vi "Create a simple numeric vi.vi"   [LabVIEW 2012]
uses:
  <vilib>/Utility/miscctls.llb/LVPointTypeDef.ctl
  <vilib>/Utility/miscctls.llb/LVBoundsTypeDef.ctl
  Scripting Tools.lvlib
types:
  T1 = typedef "LVPointTypeDef.ctl" = cluster{"Horizontal":i16, "Vertical":i16}
  T2 = typedef "LVBoundsTypeDef.ctl" = cluster{"Width":u32, "Height":u32}
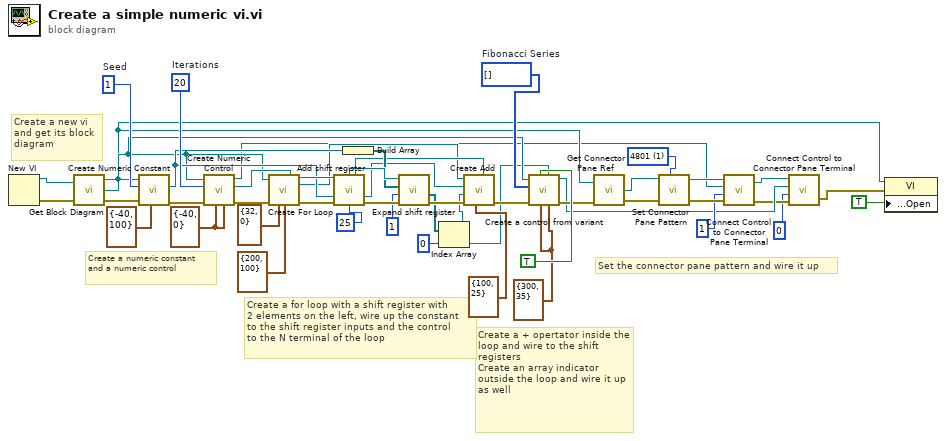
[diagram p0: block diagram]
diagram:
  w10 = u16 1 items=["4800", "4801", "4802", "4803", "4804", "4805", "4806", "4807", "4808", "4809", "4810", "4811", "4812", "4813", "4814", "4815", "4816", "4817", "4818", "4819", "4820", "4821", "4822", "4823", "4824", "4825", "4826", "4827", "4828", "4829", "4830", "4831", "4832", "4833", "4834", "4835"] ("Pattern")
  w19 = i32[] []  # Fibonacci Series
  w15 = T1 {"Horizontal"=300, "Vertical"=35} ("relative position/next to refnum")
  w16 = T1 {"Horizontal"=-40, "Vertical"=0} ("relative position/next to refnum")
  w46 = 20  # Iterations
  w43 = 1  # Seed
  # "Set the connector pane pattern and wire it up"
  # "Create a + opertator inside the loop and wire to the shift registers\nCreate an array indicator outside the loop and wire it up as well"
  # "Create a for loop with a shift register with\n2 elements on the left, wire up the constant\nto the shift register inputs and the control\nto the N terminal of the loop"
  # "Create a numeric constant\nand a numeric control"
  # "Create a new vi\nand get its block\ndiagram"
  n1 = New VI() -> (0:w47:errorcluster, 3:w48:refnum<vi>)  [unwired: 1 in, 6 out]
  n2 = call "Get Block Diagram.vi"("vi refnum in"=w48, "error in (no error)"=w47) -> ("Diagram"=w18:refnum<vi>, "vi refnum out"=w13:refnum<vi>, "error out"=w45:errorcluster)
  n3 = call "Create Numeric Constant.vi"("relative position/next to refnum"=T1 {"Horizontal"=-40, "Vertical"=100}, "error in (no error)"=w45, "Value"=w43, "Diagram"=w18) -> ("error out"=w44:errorcluster, "Output Terminal"=w32:refnum<vi>)  [unwired: 1 in, 5 out]
  n4 = call "Create Numeric Control.vi"("Terminal Position"=w16, "FP Position"=w16, "error in (no error)"=w44, "Value"=w46, "Diagram"=w18) -> ("error out"=w41:errorcluster, "Output Terminal"=w20:refnum<vi>, "Control Ref"=w7:refnum<vi>)  [unwired: 2 in, 2 out]
  n5 = call "Create For Loop.vi"("Diagram In"=w18, "Loop Count Source"=w20, "error in (no error)"=w41, "relative position/next to refnum"=T1 {"Horizontal"=32, "Vertical"=0}, "Frame Size"=T2 {"Width"=200, "Height"=100}) -> ("For Loop ref"=w37:refnum<vi>, "Diagram"=w24:refnum<vi>, "error out"=w38:errorcluster)  [unwired: 3 in, 5 out]
  n6 = call "Add shift register.vi"("Loop Reference"=w37, "Left Outside Terminal Source"=w32, "error in (no error)"=w38, "Y Positon"=u32 25) -> ("New Shift Register"=w34:refnum<vi>, "Right Inside Terminal"=w29:refnum<vi>, "Left Inside Terminal"=w28:refnum<vi>, "error out"=w35:errorcluster)  [unwired: 3 in, 5 out]
  n7 = Build Array(w32) -> (w31:refnum<vi>[])
  n8 = call "Expand shift register.vi"("error in (no error)"=w35, "New Left register count"=1, "Outer Terminal Sources"=w31, "Shift Register"=w34) -> ("error out"=w30:errorcluster, "Inner Terminals"=w27:refnum<vi>[])  [unwired: 1 in, 5 out]
  n9 = Index Array(array=w27, index=0) -> (element=w17:refnum<vi>)
  n10 = call "Create Add.vi"("Sink"=w29, "relative position/next to refnum"=T1 {"Horizontal"=100, "Vertical"=25}, "error in (no error)"=w30, "Source 2"=w17, "Source 1"=w28, "Diagram In"=w24) -> ("error out"=w25:errorcluster)  [unwired: 5 out]
  n11 = call "Create a control from variant.vi"("Terminal Position"=w15, "Terminal Source/Sink"=w17, "FP position"=w15, "Indicator?"=TRUE ("Indicator"), "error in (no error)"=w25, "Constant Data"=w19, "Diagram"=w18) -> ("error out"=w14:errorcluster, "Control Reference"=w4:refnum<vi>)  [unwired: 3 out]
  n12 = call "Get Connector Pane Ref.vi"("VI Reference"=w13, "error in (no error)"=w14) -> ("Connector Pane"=w11:refnum<vi>, "error out"=w12:errorcluster)  [unwired: 1 out]
  n13 = call "Set Connector Pane Pattern.vi"("Connector Pane"=w11, "Pattern"=w10, "error in (no error)"=w12) -> ("Connector Pane Out"=w9:refnum<vi>, "error out"=w8:errorcluster)  [unwired: 3 in, 1 out]
  n14 = call "Connect Control to Connector Pane Terminal.vi"("Connector Pane"=w9, "Control Ref"=w7, "Terminal Index"=u32 1, "error in (no error)"=w8) -> ("Connector Pane Out"=w5:refnum<vi>, "error out"=w3:errorcluster)  [unwired: 1 in]
  n15 = call "Connect Control to Connector Pane Terminal.vi"("Connector Pane"=w5, "Control Ref"=w4, "Terminal Index"=u32 0, "error in (no error)"=w3) -> ("error out"=w1:errorcluster)  [unwired: 1 in, 1 out]
  n16 = property class="VI"(reference=w13, error in=w1, "Front Panel.Open"=TRUE ("Front Panel Window:Open")) -> ()  [unwired: 2 out]
